vi "Tasten mit Text anwaehlbar markieren.vi"(7 "Anwählbar":bool, 8 "error in (no error)":errorcluster caption="Fehler (Eingang, kein Fehler)", 9 "Fehler":bool, 10 "Tastennummer":i32, 11 "Tastenreferenzen":refnum<vi>[](array[refnum])) -> (0 "error out":errorcluster caption="Fehler (Ausgang)", 3 "Tastenreferenzen (Kopie)":refnum<vi>[](array[refnum]))   [LabVIEW 2020, in "Funktionstasten.lvlib"]
doc: "Alle nicht anwählbaren Tasten grau, alle anwählbaren Tasten orange färben. Die Farbe wird durch den zugehörigen (gleicher Array-Index) Beschriftungs-String festgelegt:\nBeschriftung beginnt mit Minus-Zeichen = nicht anwählbare Taste\n\nEs sind mehr Beschriftungs-Einträge als Tasten möglich. Damit kann die Beschriftung automatisch von Enums bezogen werden, die mehr Objekte besitzen als Tasten vorhanden sind. Nur die ersten N Objekte müssen zu den N Tasten passen."
uses:
  Funktionstasten.lvlib
  Seiten/Anlagenuebersicht/VisBx Anzeige/Aktion FGV Ventile manuell schalten Crio.ctl
  Seiten/Anlagenuebersicht/VisBx Anzeige/Anlagenuebersicht.lvlib
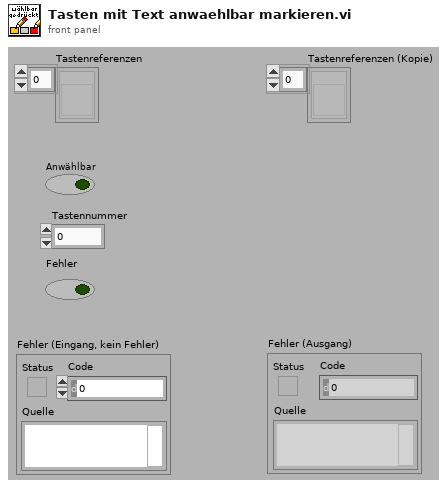
[diagram p1: front panel]
types:
  T1 = typedef "Anlagenuebersicht.lvlib/Aktion FGV Ventile manuell schalten Crio.ctl" = enum16{"lesen", "Ventile schalten", "Testbetrieb aktiv", "Testbetrieb inaktiv", "Anzeige Ventilstellung"}
  T2 = enum8{"Enabled", "Disabled", "Disabled and Grayed Out"}
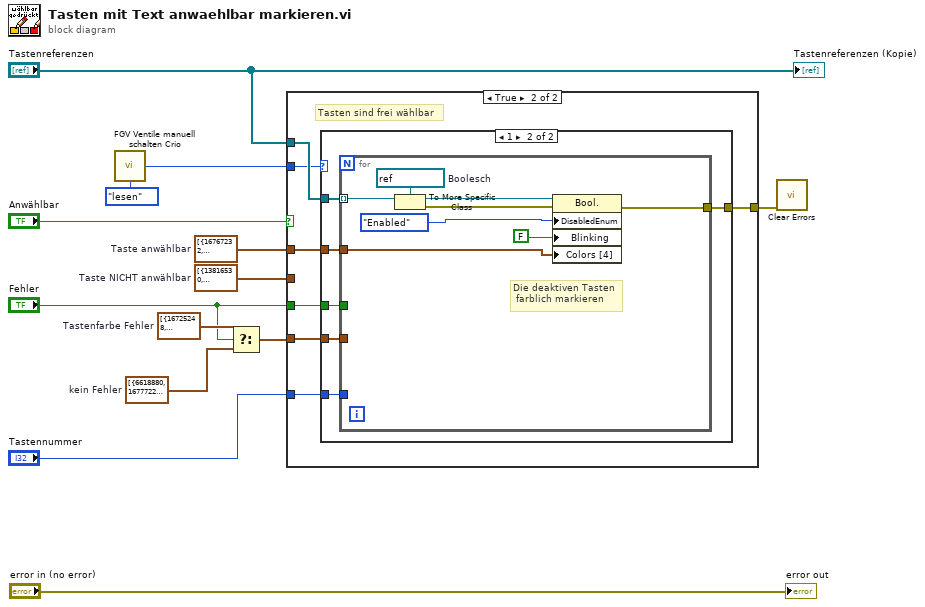
[diagram p0: block diagram]
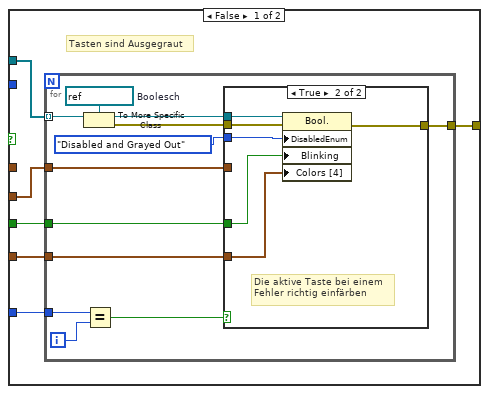
[diagram p2: hidden frame]
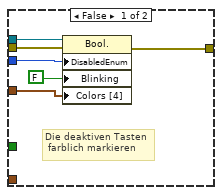
[diagram p3: hidden frame]
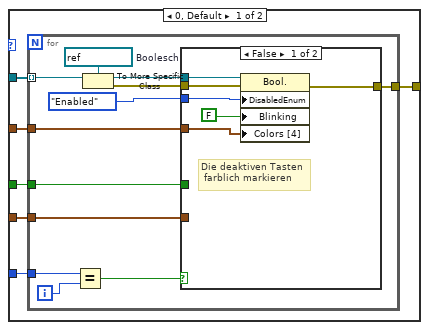
[diagram p4: hidden frame]
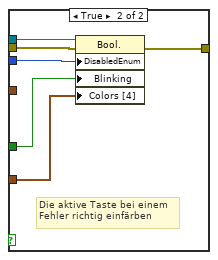
[diagram p5: hidden frame]
diagram:
  w7 = cluster{u32, u32}[] [{6618880, 16777222}]  # kein Fehler
  w11 = cluster{u32, u32}[] [{13816530, 16777222}]  # Taste NICHT anwählbar
  w8 = cluster{u32, u32}[] [{16725248, 16777222}, {16777215, 0}]  # Tastenfarbe Fehler
  w13 = cluster{u32, u32}[] [{16767232, 16777222}]  # Taste anwählbar
  n1 = call "FGV Ventile manuell schalten Crio.vi"("Aktion"=Aktion_FGV_Ventile_manuell_schalten_Crio."lesen") -> ("Betrieb"=w1:u16)  [unwired: 11 in, 3 out]
  n2 = Select(t=w8, s="Fehler", f=w7) -> (s? t:f=w6:cluster{u32, u32}[])
  n3 = case shown="True" "Anwählbar" {
    tunnel: w13 -> [_ w50]
    tunnel: "Tastenreferenzen" -> [w18 w49]
    tunnel: w11 -> [w19 _]
    tunnel: "Tastennummer" -> [w17 w47]
    tunnel: w6 -> [w16 w48]
    tunnel: "Fehler" -> [w15 w46]
    tunnel: [w14 w45] -> w3
    tunnel: w1 -> [_ w44]
    frame False {
      # "Tasten sind Ausgegraut"
      n4 = for {
        tunnel: w18 -> [w30] mode=indexing
        tunnel: w19 -> [w28]
        tunnel: w17 -> [w27]
        tunnel: w16 -> [w24]
        tunnel: w15 -> [w22]
        tunnel: [w20] -> w14
        i -> [w26]
        w31 = refnum<vi> refnum  # Boolesch
        n5 = To More Specific Class(target class=w31, reference=w30) -> (specific class reference=w29:refnum<vi>, error out=w21:errorcluster)  [unwired: 1 in]
        n6 = Equal?(x=w27, y=w26) -> (x = y?=w25:bool)
        n7 = case shown="True" w25 {
          tunnel: w29 -> [w36 w43]
          tunnel: w28 -> [w35 _]
          tunnel: w24 -> [_ w42]
          tunnel: T2."Disabled and Grayed Out" ("Deaktiviert") -> [w34 w41]
          tunnel: w22 -> [_ w40]
          tunnel: w21 -> [w32 w39]
          tunnel: [w33 w38] -> w20
          frame False {
            # "Die deaktiven Tasten\n farblich markieren"
            n8 = property class="Bool."(reference=w36, error in=w32, "DisabledEnum"=w34, "Blinking"=FALSE ("Blinkend"), "Colors [4]"=w35) -> (error out=w33:errorcluster)  [unwired: 1 out]
          }
          frame True {
            # "Die aktive Taste bei einem \nFehler richtig einfärben"
            n9 = property class="Bool."(reference=w43, error in=w39, "DisabledEnum"=w41, "Blinking"=w40, "Colors [4]"=w42) -> (error out=w38:errorcluster)  [unwired: 1 out]
          }
        }
      }
    }
    frame True {
      # "Tasten sind frei wählbar"
      n10 = case shown="1" w44 {
        tunnel: w50 -> [w56 w86]
        tunnel: w49 -> [w55 w85]
        tunnel: w48 -> [w54 w84]
        tunnel: w47 -> [w53 w83]
        tunnel: w46 -> [w52 w82]
        tunnel: [w51 w81] -> w45
        frame 0, Default {
          n11 = for {
            tunnel: w55 -> [w67] mode=indexing
            tunnel: w56 -> [w64]
            tunnel: w54 -> [w63]
            tunnel: w53 -> [w62]
            tunnel: w52 -> [w59]
            tunnel: [w57] -> w51
            i -> [w61]
            w68 = refnum<vi> refnum  # Boolesch
            n12 = Equal?(x=w62, y=w61) -> (x = y?=w60:bool)
            n13 = To More Specific Class(target class=w68, reference=w67) -> (specific class reference=w66:refnum<vi>, error out=w58:errorcluster)  [unwired: 1 in]
            n14 = case shown="False" w60 {
              tunnel: w66 -> [w73 w80]
              tunnel: w64 -> [w72 _]
              tunnel: w63 -> [_ w79]
              tunnel: T2."Enabled" ("Deaktiviert") -> [w71 w78]
              tunnel: w59 -> [_ w77]
              tunnel: w58 -> [w70 w76]
              tunnel: [w69 w75] -> w57
              frame False {
                # "Die deaktiven Tasten\n farblich markieren"
                n15 = property class="Bool."(reference=w73, error in=w70, "DisabledEnum"=w71, "Blinking"=FALSE ("Blinkend"), "Colors [4]"=w72) -> (error out=w69:errorcluster)  [unwired: 1 out]
              }
              frame True {
                # "Die aktive Taste bei einem \nFehler richtig einfärben"
                n16 = property class="Bool."(reference=w80, error in=w76, "DisabledEnum"=w78, "Blinking"=w77, "Colors [4]"=w79) -> (error out=w75:errorcluster)  [unwired: 1 out]
              }
            }
          }
        }
        frame 1 {
          n17 = for {
            tunnel: w85 -> [w93] mode=indexing
            tunnel: w86 -> [w90]
            tunnel: w84 -> [_]
            tunnel: w83 -> [_]
            tunnel: w82 -> [_]
            tunnel: [w88] -> w81
            w94 = refnum<vi> refnum  # Boolesch
            # "Die deaktiven Tasten\n farblich markieren"
            n18 = To More Specific Class(target class=w94, reference=w93) -> (specific class reference=w92:refnum<vi>, error out=w89:errorcluster)  [unwired: 1 in]
            n19 = property class="Bool."(reference=w92, error in=w89, "DisabledEnum"=T2."Enabled" ("Deaktiviert"), "Blinking"=FALSE ("Blinkend"), "Colors [4]"=w90) -> (error out=w88:errorcluster)  [unwired: 1 out]
          }
        }
      }
    }
  }
  n20 = call <vilib>:"Clear Errors.vi"("error in (no error)"=w3) -> ()  [unwired: 5 in, 2 out]
  "error out" <- "error in (no error)"
  "Tastenreferenzen (Kopie)" <- "Tastenreferenzen"
